vi "LVObject to JSON.vi"(5 "enable LabVIEW extensions? (T)":bool=TRUE, 6 "Pretty Print?":bool, 7 "Demo LVClass Serializer in":refnum<class "Demo LVClass Serializer.lvclass">, 8 "error in (no error)":errorcluster, 10 "Object":refnum<class>) -> (0 "error out":errorcluster, 2 "<JSON>Object":string)   [LabVIEW 2019, in "Demo LVClass Serializer.lvclass"]
doc: "Convert Object of a LabVIEW Class to a JSON representation.\n\nThis demonstration converts to an XML representation in a JSON String."
uses:
  Demo LVClass Serializer.lvclass
  vi.lib/JDP Science/JSONtext/JSONtext.lvlib
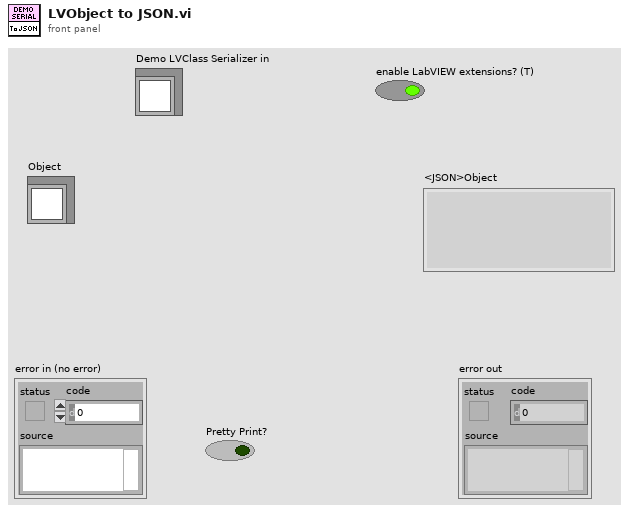
[diagram p1: front panel]
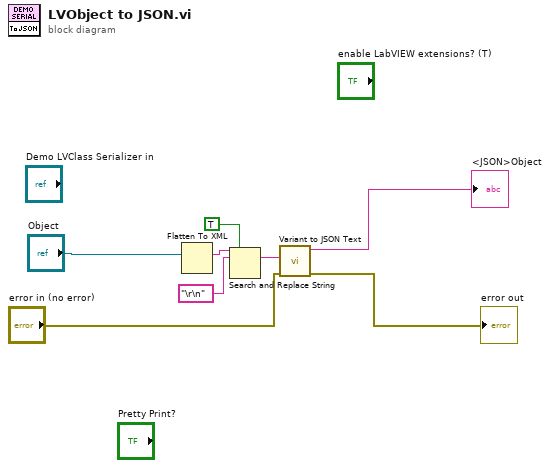
[diagram p0: block diagram]
diagram:
  n1 = Flatten To XML(anything="Object") -> (xml string=w2:string)
  n2 = Search and Replace String(replace all?=TRUE ("replace all? (F)"), input string=w2, search string="\r\n" ("xml string")) -> (result string=w4:string)  [unwired: 5 in, 3 out]
  n3 = call "Variant to JSON Text.vi"("error in (no error)"="error in (no error)", "Variant"=w4) -> ("error out"=→"error out":errorcluster, "<JSON>"=→"<JSON>Object":string)  [unwired: 7 in, 1 out]
